vi "Draw Layers.vi"(7 "Active User Layer Data []":i32[](array[numeric]), 8 "#Active Layer":i32, 9 "#User Layer":i32, 10 "Highlighted? (F)":bool, 11 "Layers":refnum<class "Layer.lvclass">[](array[class])) -> (3 "Picture":picture)   [LabVIEW 2020, in "lv_icon.lvlib"]
doc: "Merges all User Layers based on their information (Origin and Type)."
uses:
  resource/plugins/lv_icon.lvlib
  Classes/Layer/Layer.lvclass
  LabVIEW Icon API.lvlib
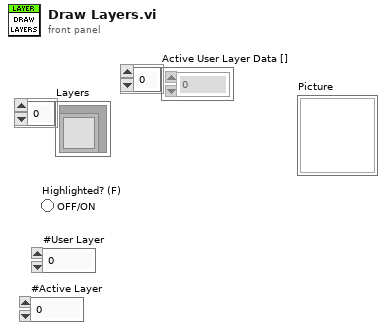
[diagram p1: front panel]
types:
  T1 = typedef "Layer.ctl" = cluster{"LayerIcon":picture, "LayerName":string, "Opacity":u8, "Visibility?":bool}
  T2 = typedef "LVPoint32TypeDef.ctl" = cluster{"Horizontal":i32, "Vertical":i32}
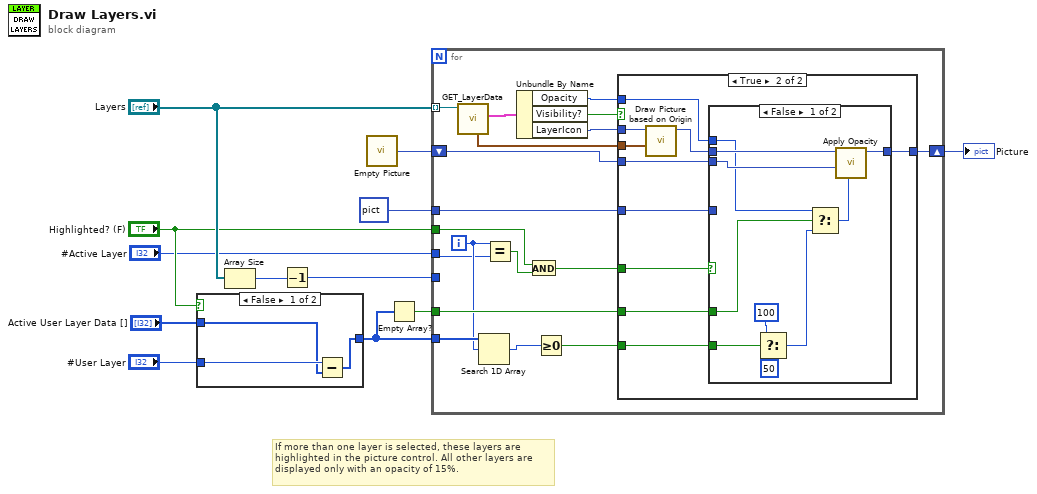
[diagram p0: block diagram]
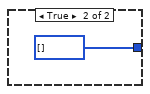
[diagram p2: hidden frame]
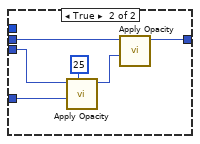
[diagram p4: hidden frame]
diagram:
  # "If more than one layer is selected, these layers are\nhighlighted in the picture control. All other layers are\ndisplayed only with an opacity of 15%."
  n1 = case shown="False" "Highlighted? (F)" {
    tunnel: [w15 i32[] [] ("Active Data []")] -> w3
    tunnel: "#User Layer" -> [w14 _]
    tunnel: "Active User Layer Data []" -> [w13 _]
    frame False {
      n2 = Subtract(x=w14, y=w13) -> (x-y=w15:i32[])
    }
    frame True {
    }
  }
  n3 = Array Size(array="Layers") -> (size(s)=w5:i32)
  n4 = Decrement(x=w5) -> (x-1=w6:i32)
  n5 = call "Empty Picture"() -> ("empty picture"=w10:picture)
  n6 = Empty Array?(array=w3) -> (empty?=w7:bool)
  n7 = for {
    shift-right: [w31] -> w12
    shift-left: w10 -> [w32]
    tunnel: "Layers" -> [w29] mode=indexing
    tunnel: picture data[5B] ("new picture") -> [w26]
    tunnel: w6 -> [_]
    tunnel: "Highlighted? (F)" -> [w25]
    tunnel: w3 -> [w23]
    tunnel: w7 -> [w22]
    tunnel: "#Active Layer" -> [w18]
    i -> [w19]
    n8 = call-dynamic "GET_LayerData.vi"("Layer.lvclass in"=w29) -> ("Data"=w28:T1, "Origin"=w27:T2)  [unwired: 1 in, 8 out]
    n9 = Search 1D Array(1D array=w23, element=w19) -> (index of element=w21:i32)  [unwired: 1 out]
    n10 = Equal?(x=w19, y=w18) -> (x = y?=w17:bool)
    n11 = Unbundle By Name(w28) -> ("Opacity"=w33:u8, "Visibility?"=w34:bool, "LayerIcon"=w30:picture)
    n12 = And(x=w25, y=w17) -> (x .and. y?=w24:bool)
    n13 = Greater Or Equal To 0?(x=w21) -> (x >= 0?=w20:bool)
    n14 = case shown="True" w34 {
      tunnel: w33 -> [_ w45]
      tunnel: w32 -> [w35 w44]
      tunnel: [w35 w43] -> w31
      tunnel: w30 -> [_ w42]
      tunnel: w27 -> [_ w41]
      tunnel: w26 -> [_ w38]
      tunnel: w24 -> [_ w39]
      tunnel: w22 -> [_ w37]
      tunnel: w20 -> [_ w36]
      frame False {
      }
      frame True {
        n15 = call "Draw Picture based on Origin.vi"("Origin"=w41, "LayerIcon in"=w42) -> ("LayerIcon out"=w40:picture)  [unwired: 1 in, 8 out]
        n16 = case shown="False" w39 {
          tunnel: w45 -> [w52 _]
          tunnel: w44 -> [w55 w56]
          tunnel: [w54 w58] -> w43
          tunnel: w40 -> [w53 w59]
          tunnel: w38 -> [_ w57]
          tunnel: w37 -> [w51 _]
          tunnel: w36 -> [w49 _]
          frame False {
            n17 = Select(t=u8 100 ("f"), s=w49, f=u8 50) -> (s? t:f=w46:u8)
            n18 = Select(t=w52, s=w51, f=w46) -> (s? t:f=w50:u8)
            n19 = call "Apply Opacity.vi"("% (100)"=w50, "Bottom"=w55, "Top"=w53) -> ("new picture"=w54:picture)  [unwired: 8 out]
          }
          frame True {
            n20 = call "Apply Opacity.vi"("% (100)"=u8 25, "Bottom"=w57, "Top"=w56) -> ("new picture"=w60:picture)  [unwired: 8 out]
            n21 = call "Apply Opacity.vi"("Bottom"=w60, "Top"=w59) -> ("new picture"=w58:picture)  [unwired: 1 in, 8 out]
          }
        }
      }
    }
  }
  "Picture" <- w12
